vi "Dequeue Timed Out.vi"(4 "Priority In":i32, 6 "Timed Out":bool, 7 "Wait Prior":refnum<queue>, 8 "error in (no error)":errorcluster, 9 "Message In":refnum<class "Message.lvclass">, 10 "Wait Msg":refnum<queue>, 11 "Ref":refnum<data-value>) -> (0 "error out":errorcluster, 1 "Priority":i32, 2 "Message":refnum<class "Message.lvclass">, 3 "Really Timed Out":bool)   [LabVIEW 2020, in "Artifex.lvlib" / "Priority Message Queue.lvclass"]
uses:
  Priority Message Queue.lvclass
  Message/Message.lvclass
  Ref Data.ctl
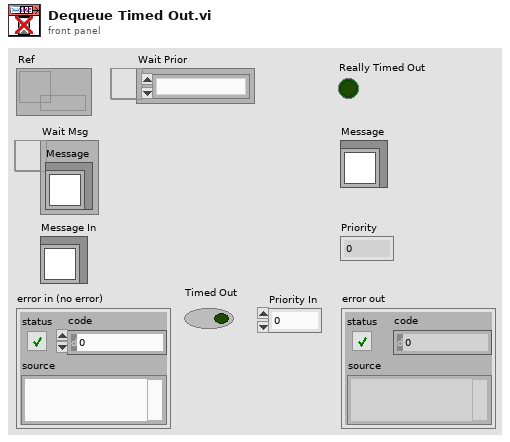
[diagram p1: front panel]
types:
  T1 = typedef "Artifex.lvlib/Priority Message Queue.lvclass/Ref Data.ctl" = cluster{"# Waiting":u32, "Buffers":refnum<queue>[], "Wait Msg":refnum<queue>, "Wait Prior":refnum<queue>}
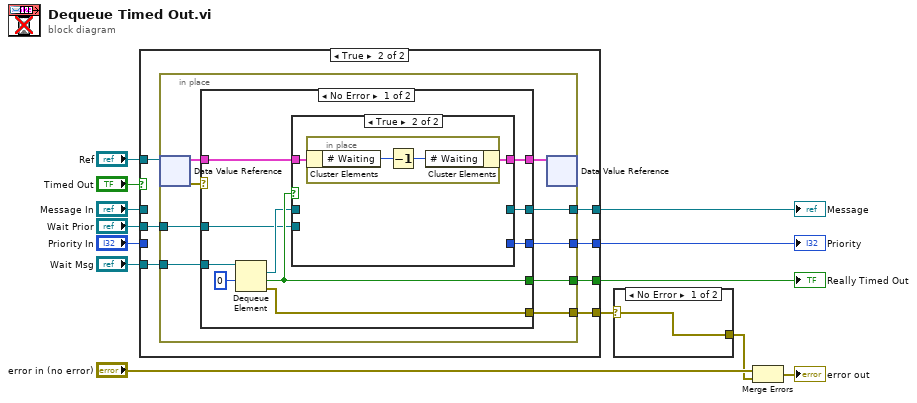
[diagram p0: block diagram]
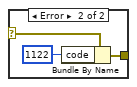
[diagram p2: hidden frame]
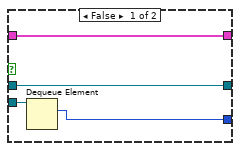
[diagram p4: hidden frame]
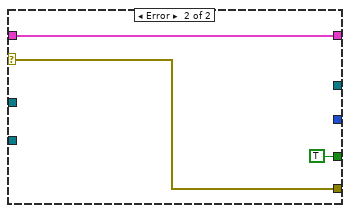
[diagram p5: hidden frame]
diagram:
  n1 = case shown="True" "Timed Out" {
    selector: "Timed Out" -> [w14 _]
    tunnel: "Message In" -> [w16 _]
    tunnel: [w16 w19] -> w11
    tunnel: [w15 w18] -> w10
    tunnel: "Priority In" -> [w15 _]
    tunnel: [w14 w21] -> w8
    tunnel: "Ref" -> [_ w23]
    tunnel: "Wait Msg" -> [_ w22]
    tunnel: "Wait Prior" -> [_ w20]
    tunnel: [_ w17] -> w4
    frame False {
    }
    frame True {
      n2 = in-place {
        in-place-border: w22 -> [w30]
        in-place-border: [w29] -> w21
        in-place-border: w20 -> [w28]
        in-place-border: [w27] -> w19
        in-place-border: [w26] -> w18
        in-place-border: [w24] -> w17
        n3 = in-place-dvr #1(w23) -> (w32:T1, w31:errorcluster)
        n4 = case shown="No Error" w31 {
          selector: w31 -> [_ w51]
          tunnel: w32 -> [w35 w53]
          tunnel: w30 -> [w42 _]
          tunnel: [w40 TRUE ("timed out?")] -> w29
          tunnel: w28 -> [w37 _]
          tunnel: [w38 _] -> w27
          tunnel: [w36 _] -> w26
          tunnel: [w34 w53] -> w25
          tunnel: [w33 w51] -> w24
          frame No Error {
            n5 = Dequeue Element(queue=w42, timeout in ms (-1)=0) -> (element=w39:refnum<class "Message.lvclass">, timed out?=w40:bool, error out=w33:errorcluster)  [unwired: 1 in, 1 out]
            n6 = case shown="True" w40 {
              tunnel: w39 -> [w46 _]
              tunnel: [w46 _] -> w38
              tunnel: w37 -> [w45 _]
              tunnel: [w44 _] -> w36
              tunnel: w35 -> [w43 w48]
              tunnel: [w43 w47] -> w34
              frame False {
                n7 = Dequeue Element(queue=w45) -> (element=w44:i32)  [unwired: 2 in, 3 out]
              }
              frame True {
                n8 = in-place {
                  n9 = in-place-cluster #2(w48) -> ("# Waiting"=w50:u32)
                  n10 = Decrement(x=w50) -> (x-1=w49:u32)
                  n11 = in-place-cluster #2("# Waiting"=w49) -> (w47:T1)
                }
              }
            }
          }
          frame Error {
          }
        }
        n12 = in-place-dvr #1(w25) -> ()  [unwired: 2 out]
      }
    }
  }
  "Really Timed Out" <- w8
  "Message" <- w11
  "Priority" <- w10
  n13 = case shown="No Error" w4 {
    selector: w4 -> [w54 w57]
    tunnel: [w54 w55] -> w2
    frame No Error {
    }
    frame Error {
      n14 = Bundle By Name(cluster=w57, "code"=1122) -> (w55:errorcluster)
    }
  }
  n15 = Merge Errors("error in (no error)", w2) -> (→"error out":errorcluster)
